vi "motor_startup.vi"() -> ()   [LabVIEW 2015]
panel:
  out "error out":errorcluster
  in  "error in (no error)":errorcluster
  in  "Motor #":u8
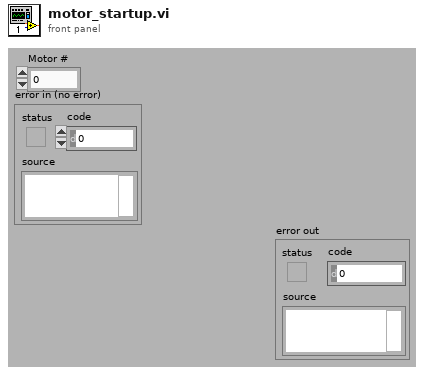
[diagram p1: front panel]
types:
  T1 = enum16{"POL (0)", "CPL (1)", "HLT (2)", "STP (3)", "RST (4)", "RVN (5)", "RPB (6)", "CLP (8)", "SDL (9)", "RUN (10)", "WRI (11)", "RRG (12)", "SPR (13)", "LPR (14)", "VMI (15)", "SSP (17)", "SSE (18)", "RIS (20)", "RIO (21)", "IMW (25)", "END (128)", "MAV (134)", "MRV (135)", "JRE (137)", "WCL (138)", "WCW (139)", "DLY (140)", "WDL (141)", "GCL (142)", "GOP (143)", "ZTG (144)", "ZTP (145)", "TTP (146)", "CME (147)", "CTC (148)", "TQL (149)", "AHC (150)", "ERL (151)", "OLP (152)", "WRP (154)", "IDT (155)", "LRP (156)", "VMP (159)", "RAV (160)", "RRV (161)", "JMP (162)", "JOI (162)", "CIS (163)", "CKS (164)", "CLC (165)", "KMC (167)", "MCT (168)", "FLC (169)", "EEM (170)", "DDB (171)", "DEM (171)", "PAC (172)", "ADL (173)", "BRT (174)", "MAT (176)", "MRT (177)", "RAT (178)", "RRT (179)", "SSD (180)", "KMR (181)", "KED (182)", "KDD (183)", "DIR (184)", "PRO (185)", "SIF (186)", "EDL (187)", "CIO (188)", "MDS (189)", "MDC (190)", "MDT (191)", "SEE (192)", "ARI (193)", "WBS (194)", "SCF (195)", "RSM (196)", "RLM (197)", "RSN (198)", "RLN (199)", "PCL (201)", "PCI (201)", "PRT (202)", "PRI (202)", "WBE (204)", "SOB (205)", "COB (206)", "ACR (207)", "PLR (208)", "CAI (211)", "LVT (212)", "OVT (213)", "MTT (214)", "CLC (215)", "PIM (216)", "VIM (217)", "TIM (218)", "AHM (219)", "SSL (221)", "TRU (222)", "RSD (223)", "EMT (225)", "DMT (226)", "EMD (227)", "DMD (228)", "HSM (229)", "AHD (230)", "PCM (231)", "PCG (232)", "XRV (233)", "XAV (234)", "XRT (235)", "XAT (236)", "GOC (237)", "JNA (238)", "JOR (239)", "PMC (240)", "PMV (241)", "PMX (242)", "DLC (243)", "SLC (244)", "PCP (245)", "ATR (248)", "PMO (249)", "JAN (250)", "EDH (251)", "DIF (252)", "IMS (253)", "IMQ (254)"}
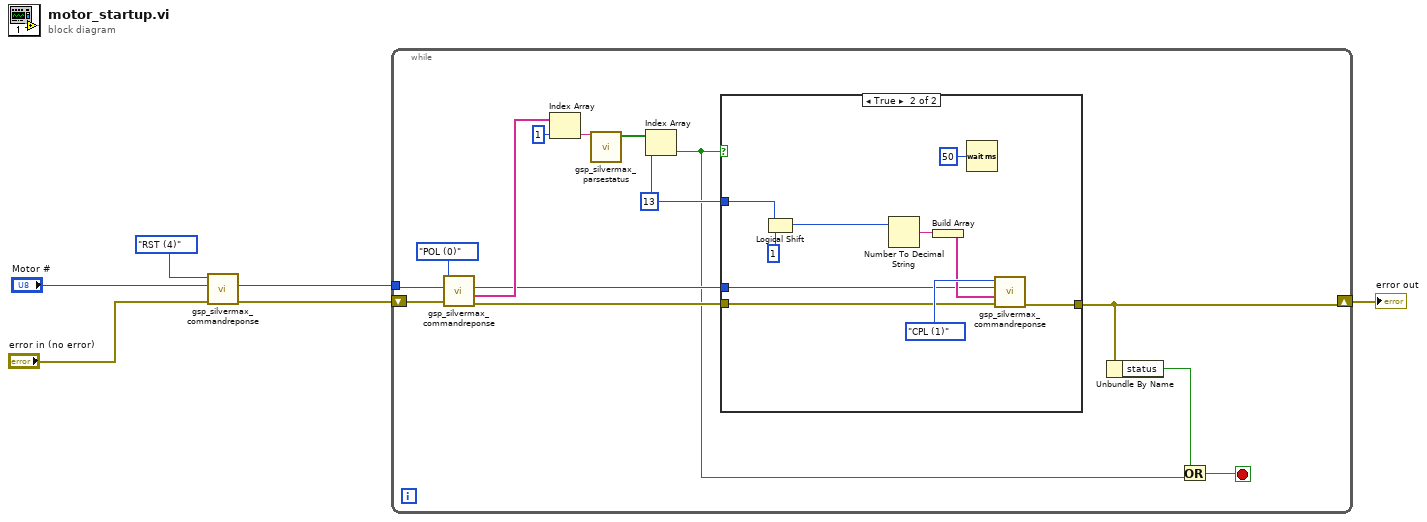
[diagram p0: block diagram]
diagram:
  n1 = call "gsp_silvermax_commandreponse.vi"("error in (no error)"="error in (no error)", "Motor #"="Motor #", "Command"=T1."RST (4)") -> ("error out"=w2:errorcluster, "Motor # dup"=w3:u8)  [unwired: 1 in, 2 out]
  n2 = while {
    tunnel: w3 -> [w17]
    shift-right: [w8] -> w1
    shift-left: w2 -> [w18]
    stop <- w20 stop-if-true
    w10 = 13 ("index")
    n3 = call "gsp_silvermax_commandreponse.vi"("error in (no error)"=w18, "Motor #"=w17, "Command"=T1."POL (0)") -> ("error out"=w12:errorcluster, "Parameter Array"=w16:string[], "Motor # dup"=w11:u8)  [unwired: 1 in, 1 out]
    n4 = Index Array(array=w16, index=1) -> (element=w14:string)
    n5 = call "gsp_silvermax_parsestatus.vi"("Status Word in Hex"=w14) -> ("Boolean Array"=w13:bool[])  [unwired: 6 in]
    n6 = Index Array(array=w13, index=w10) -> (element=w7:bool)
    n7 = case shown="True" w7 {
      tunnel: w12 -> [w21 w26]
      tunnel: w11 -> [_ w25]
      tunnel: w10 -> [_ w24]
      tunnel: [w21 w23] -> w8
      frame False {
      }
      frame True {
        n8 = Logical Shift(y=w24, x=u16 1) -> (x << y=w27:u16)
        n9 = Number To Decimal String(number=w27) -> (decimal integer string=w30:string)  [unwired: 1 in]
        n10 = Build Array(w30) -> (w28:string[])
        n11 = Wait (ms)(milliseconds to wait=u32 50) -> ()  [unwired: 1 out]
        n12 = call "gsp_silvermax_commandreponse.vi"("error in (no error)"=w26, "Parameters (none)"=w28, "Motor #"=w25, "Command"=T1."CPL (1)") -> ("error out"=w23:errorcluster)  [unwired: 3 out]
      }
    }
    n13 = Unbundle By Name(w8) -> ("status"=w9:bool)
    n14 = Or(x=w9, y=w7) -> (x .or. y?=w20:bool)
  }
  "error out" <- w1
